vi "选择排空留样瓶对话框.vi"() -> (2 "布尔":bool=TRUE, 3 "选择留样瓶 2":u16)   [LabVIEW 2016, in "超标留样集成.lvlib" / "德润DR803L超标留样.lvlib"]
uses:
  <vilib>/Utility/miscctls.llb/LVPointTypeDef.ctl
panel:
  in  "取消":bool
  in  "确定":bool
  in  "选择留样瓶":u16
  # "请选择留样瓶号0~12(0:排空所有瓶)"
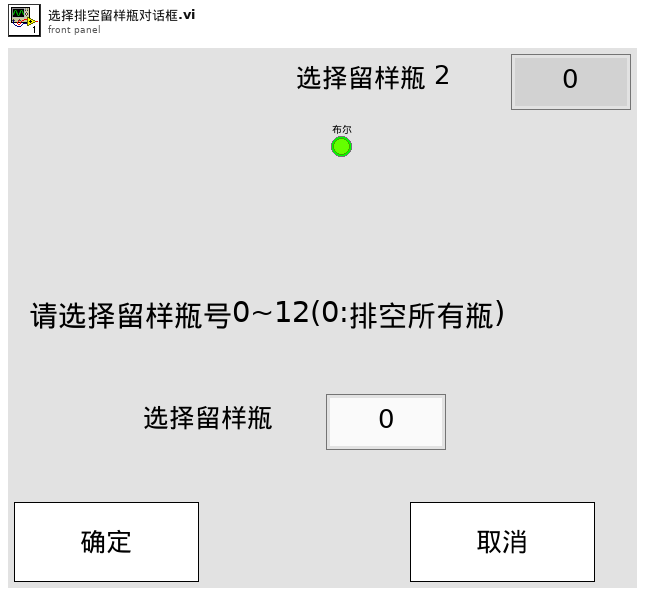
[diagram p1: front panel]
types:
  T1 = typedef "LVPointTypeDef.ctl" = cluster{"Horizontal":i16, "Vertical":i16}
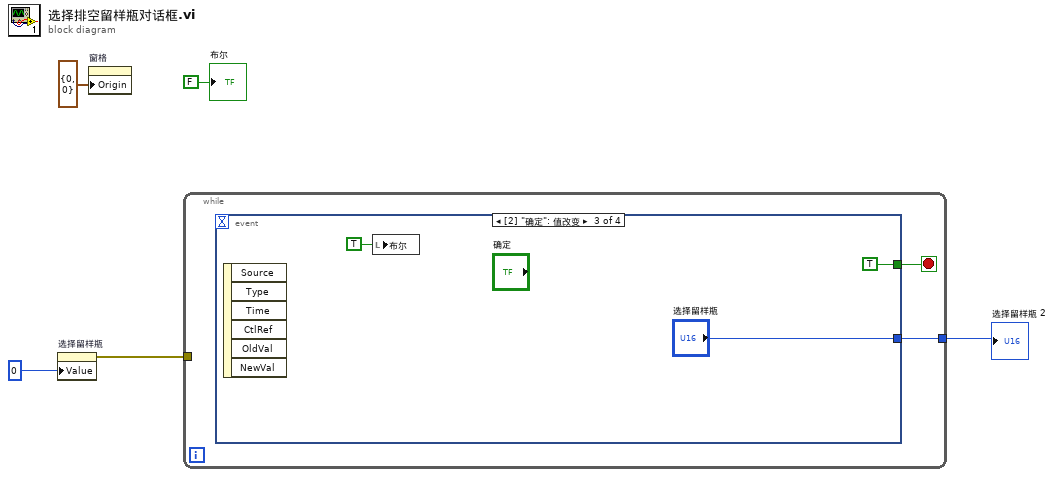
[diagram p0: block diagram]
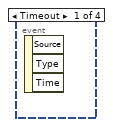
[diagram p2: hidden frame]
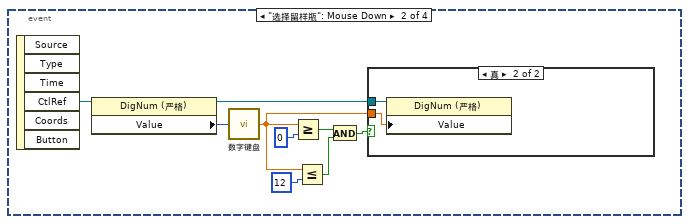
[diagram p3: hidden frame]
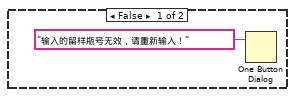
[diagram p4: hidden frame]
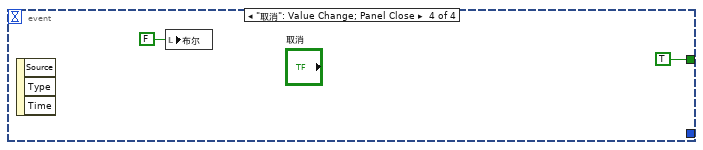
[diagram p5: hidden frame]
diagram:
  n1 = property on="选择留样瓶" class="DigNum (严格)"("Value"=u16 0 ("选择留样瓶")) -> (error out=w2:errorcluster)  [unwired: 2 in, 1 out]
  n2 = property on="窗格" class="Pane"("Origin"=T1 {"Horizontal"=0, "Vertical"=0} ("原点")) -> ()  [unwired: 2 in, 2 out]
  n3 = while {
    tunnel: w2 -> [_]
    tunnel: [w6] -> w1
    stop <- w7 stop-if-true
    n4 = event shown="[2] \"确定\": 值改变" {
      selector: _ -> [_ _ _ _]
      dyn-events: _ -> [_ _ _ _]
      timeout: _ -> [_ _ _ _]
      tunnel: [_ _ TRUE TRUE] -> w7
      tunnel: [_ _ "选择留样瓶" _] -> w6
      event Timeout {
        n5 = event-data() -> ()  [unwired: 1 in, 3 out]
      }
      event "选择留样瓶": Mouse Down {
        n6 = event-data() -> ("CtlRef"=w16:refnum<vi>)  [unwired: 1 in, 5 out]
        n7 = property class="DigNum (严格)"(reference=w16) -> (reference out=w15:refnum<vi>, "Value"=w14:u16)  [unwired: 1 in, 1 out]
        n8 = call "数字键盘.vi"("OldNumber"=w14) -> ("NewNumber"=w12:sgl)
        n9 = Greater Or Equal?(x=w12, y=u16 0) -> (x >= y?=w10:bool)
        n10 = Less Or Equal?(x=w12, y=u16 12) -> (x <= y?=w9:bool)
        n11 = And(x=w10, y=w9) -> (x .and. y?=w8:bool)
        n12 = case shown="真" w8 {
          tunnel: w15 -> [_ w19]
          tunnel: w12 -> [_ w18]
          frame False {
            n13 = One Button Dialog(message="输入的留样瓶号无效，请重新输入！" ("消息")) -> ()  [unwired: 1 in, 1 out]
          }
          frame True {
            n14 = property class="DigNum (严格)"(reference=w19, "Value"=w18) -> ()  [unwired: 1 in, 2 out]
          }
        }
      }
      event "确定": Value Change {
        n15 = event-data() -> ()  [unwired: 1 in, 6 out]
        n16 = local write "布尔"(TRUE ("布尔")) -> ()
      }
      event "取消": Value Change; Panel Close {
        n17 = event-data() -> ()  [unwired: 1 in, 3 out]
        n18 = local write "布尔"(FALSE ("布尔")) -> ()
      }
    }
  }
  "选择留样瓶 2" <- w1
  "布尔" <- FALSE ("布尔")
